vi "Nearest Integers for Direction.vi"(10 "Tolerance":dbl, 11 "Direction":dbl[](array[numeric])=[1.0, 0.0, 0.0]) -> (2 "Sugested Factor":dbl, 3 "Nearest Integer Directions":dbl[](array[numeric])=[1.0, 0.0, 0.0])   [LabVIEW 2010]
panel:
  out "System XY Graph":cluster{dbl[], dbl[]}[](graph)
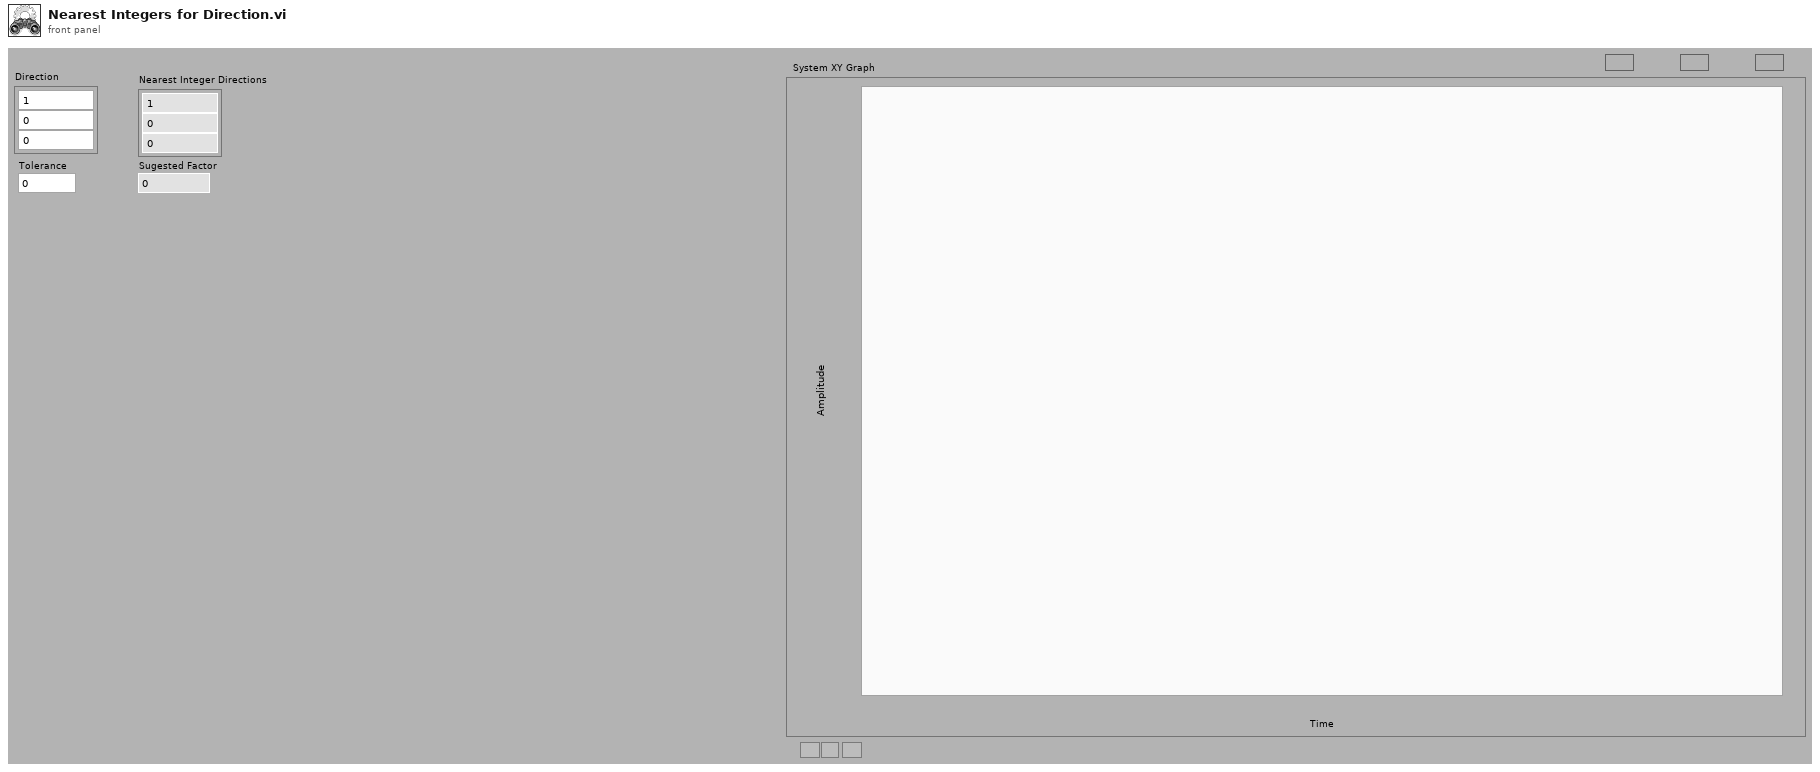
[diagram p1: front panel]
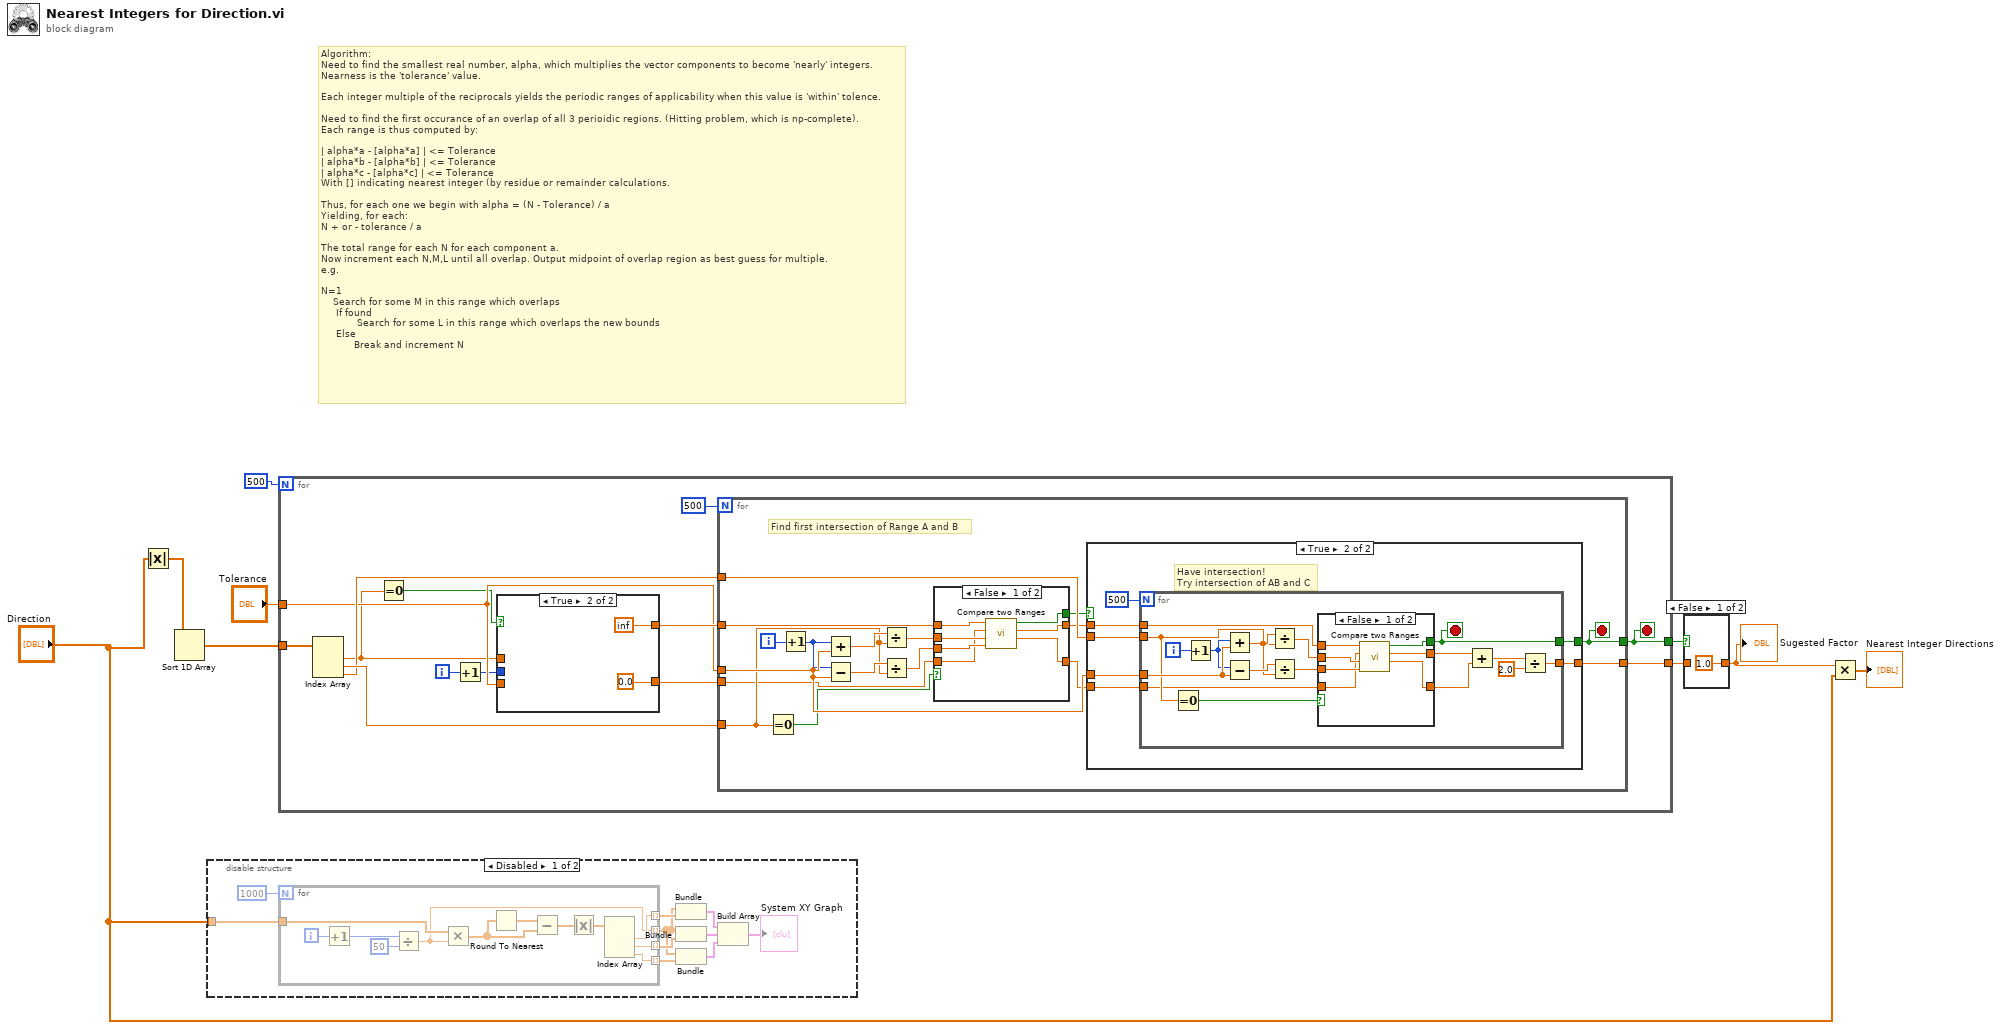
[diagram p0: block diagram]
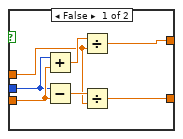
[diagram p4: hidden frame]
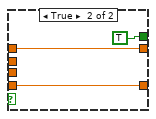
[diagram p5: hidden frame]
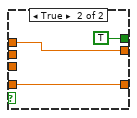
[diagram p7: hidden frame]
diagram:
  # "Algorithm:\nNeed to find the smallest real number, alpha, which multiplies the vector components to become 'nearly' integers.\nNearness is the 'tolerance' value.\n\nEach integer multiple of the reciprocals yields the periodic ranges of applicability when this value is 'within' tolence.\n\nNeed to find the first occurance of an overlap of all 3 perioidic regions. (Hitting problem, which is np-complete).\nEach range is thus computed by:\n\n| alpha*a - [alpha*a] | <= Tolerance\n| alpha*b - [alpha*b] | <= Tolerance\n| alpha*c - [alpha*c] | <= Tolerance\nWith [] indicating nearest integer (by residue or remainder calculations.\n\nThus, for each one we begin with alpha = (N - Tolerance) / a\nYielding, for each:\nN + or - tolerance / a\n\nThe total range for each N for each component a.\nNow increment each N,M,L until all overlap. Output midpoint of overlap region as best guess for multiple.\ne.g.\n\nN=1\n    Search for some M in this range which overlaps\n     If found\n            Search for some L in this range which overlaps the new bounds\n     Else\n           Break and increment N"
  n1 = Absolute Value(x="Direction") -> (abs(x)=w1:dbl[])
  n2 = Sort 1D Array(array=w1) -> (sorted array=w3:dbl[])
  n3 = disable-structure shown="Disabled" {
    disable-tunnel: "Direction" -> [w19 _]
    frame Disabled {
      n4 = for {
        N: 1000 -> [_]
        tunnel: w19 -> [w26]
        tunnel: [w23] -> w17 mode=indexing
        tunnel: [w22] -> w15 mode=indexing
        tunnel: [w21] -> w16 mode=indexing
        tunnel: [w20] -> w14 mode=indexing
        i -> [w29]
        n5 = Increment(x=w29) -> (x+1=w28:i32)
        n6 = Divide(x=w28, y=50) -> (x/y=w20:dbl)
        n7 = Multiply(x=w26, y=w20) -> (x*y=w25:dbl[])
        n8 = Round To Nearest(number=w25) -> (nearest integer value=w30:dbl[])
        n9 = Subtract(x=w30, y=w25) -> (x-y=w31:dbl[])
        n10 = Absolute Value(x=w31) -> (abs(x)=w24:dbl[])
        n11 = Index Array(array=w24) -> (element #1=w23:dbl, element #2=w21:dbl, element #3=w22:dbl)  [unwired: 3 in]
      }
      n12 = Bundle(w14, w17) -> (w13:cluster{dbl[], dbl[]})  [unwired: 1 in]
      n13 = Bundle(w14, w16) -> (w12:cluster{dbl[], dbl[]})  [unwired: 1 in]
      n14 = Bundle(w14, w15) -> (w11:cluster{dbl[], dbl[]})  [unwired: 1 in]
      n15 = Build Array(w13, w12, w11) -> (→"System XY Graph":cluster{dbl[], dbl[]}[])
    }
    frame Enabled {
    }
  }
  n16 = for {
    N: 500 -> [_]
    tunnel: w3 -> [w43]
    tunnel: "Tolerance" -> [w38]
    tunnel: [w37] -> w9
    tunnel: [w36] -> w8
    i -> [w44]
    stop <- w37 stop-if-true
    n17 = Index Array(array=w43) -> (element #1=w33:dbl, element #2=w40:dbl, element #3=w39:dbl)  [unwired: 3 in]
    n18 = Equal To 0?(x=w33) -> (x = 0?=w32:bool)
    n19 = Increment(x=w44) -> (x+1=w35:i32)
    n20 = case shown="True" w32 {
      tunnel: [w49 inf] -> w42
      tunnel: [w48 0.0] -> w41
      tunnel: w38 -> [w47 _]
      tunnel: w35 -> [w46 _]
      tunnel: w33 -> [w45 _]
      frame False {
        n21 = Add(x=w46, y=w47) -> (x+y=w51:dbl)
        n22 = Subtract(x=w46, y=w47) -> (x-y=w50:dbl)
        n23 = Divide(x=w51, y=w45) -> (x/y=w49:dbl)
        n24 = Divide(x=w50, y=w45) -> (x/y=w48:dbl)
      }
      frame True {
      }
    }
    n25 = for {
      N: 500 -> [_]
      tunnel: w42 -> [w55]
      tunnel: w41 -> [w56]
      tunnel: w40 -> [w62]
      tunnel: w39 -> [w67]
      tunnel: w38 -> [w66]
      tunnel: [w65] -> w37
      tunnel: [w64] -> w36
      i -> [w68]
      stop <- w65 stop-if-true
      # "Find first intersection of Range A and B"
      n26 = Equal To 0?(x=w62) -> (x = 0?=w54:bool)
      n27 = Increment(x=w68) -> (x+1=w63:i32)
      n28 = Add(x=w63, y=w66) -> (x+y=w69:dbl)
      n29 = Subtract(x=w63, y=w66) -> (x-y=w70:dbl)
      n30 = Divide(x=w69, y=w62) -> (x/y=w60:dbl)
      n31 = Divide(x=w70, y=w62) -> (x/y=w61:dbl)
      n32 = case shown="False" w54 {
        tunnel: w61 -> [w77 _]
        tunnel: w60 -> [w76 _]
        tunnel: [w75 w79] -> w59
        tunnel: [w74 TRUE ("In Range")] -> w58
        tunnel: [w73 w80] -> w57
        tunnel: w56 -> [w72 w79]
        tunnel: w55 -> [w71 w80]
        frame False {
          n33 = call "Compare two Ranges.vi"("Lower 2"=w77, "Upper 2"=w76, "Lower 1"=w72, "Upper 1"=w71) -> ("Lower"=w75:dbl, "Upper"=w73:dbl, "In Range"=w74:bool)  [unwired: 5 in]
        }
        frame True {
        }
      }
      n34 = case shown="True" w58 {
        tunnel: w57 -> [_ w86]
        tunnel: w59 -> [_ w85]
        tunnel: w67 -> [_ w87]
        tunnel: w66 -> [_ w84]
        tunnel: [_ w83] -> w65
        tunnel: [_ w82] -> w64
        frame False {
        }
        frame True {
          # "Have intersection!\nTry intersection of AB and C"
          n35 = for {
            N: 500 -> [_]
            tunnel: w87 -> [w96]
            tunnel: w86 -> [w89]
            tunnel: w85 -> [w88]
            tunnel: w84 -> [w101]
            tunnel: [w95] -> w83
            tunnel: [w98] -> w82
            i -> [w102]
            stop <- w95 stop-if-true
            n36 = Equal To 0?(x=w96) -> (x = 0?=w90:bool)
            n37 = Increment(x=w102) -> (x+1=w97:i32)
            n38 = Add(x=w97, y=w101) -> (x+y=w104:dbl)
            n39 = Subtract(x=w97, y=w101) -> (x-y=w103:dbl)
            n40 = Divide(x=w104, y=w96) -> (x/y=w92:dbl)
            n41 = Divide(x=w103, y=w96) -> (x/y=w91:dbl)
            n42 = case shown="False" w90 {
              tunnel: w91 -> [w111 _]
              tunnel: w92 -> [w110 _]
              tunnel: [w109 w113] -> w93
              tunnel: [w108 TRUE ("In Range")] -> w95
              tunnel: [w107 w114] -> w94
              tunnel: w88 -> [w106 w113]
              tunnel: w89 -> [w105 w114]
              frame False {
                n43 = call "Compare two Ranges.vi"("Lower 2"=w111, "Upper 2"=w110, "Lower 1"=w106, "Upper 1"=w105) -> ("Lower"=w109:dbl, "Upper"=w107:dbl, "In Range"=w108:bool)  [unwired: 5 in]
              }
              frame True {
              }
            }
            n44 = Add(x=w94, y=w93) -> (x+y=w99:dbl)
            n45 = Divide(x=w99, y=2.0) -> (x/y=w98:dbl)
          }
        }
      }
    }
  }
  n46 = case shown="False" w9 {
    tunnel: w8 -> [_ w116]
    tunnel: [1.0 w116] -> w7
    frame False {
    }
    frame True {
    }
  }
  "Sugested Factor" <- w7
  n47 = Multiply(x=w7, y="Direction") -> (x*y=→"Nearest Integer Directions":dbl[])
